vi "Command Drive Distance.vi"(6 "Timeout":dbl=3.0, 8 "Speed":dbl=0.4, 9 "Heading":dbl, 10 "Distance(Feet)":dbl=14.0, 11 "Startup":bool) -> (0 "Angular":dbl, 1 "Reinit":bool, 2 "Linear":dbl, 3 "Completed":bool=TRUE)   [LabVIEW 2019]
uses:
  Command_Execution_State.ctl
  Globals/Sensor_Values.vi
panel:
  in  "Turn Gain":dbl=0.09
  in  "Distance Gain":dbl=0.01
  # "Alpha .06"
  # "Beta .1"
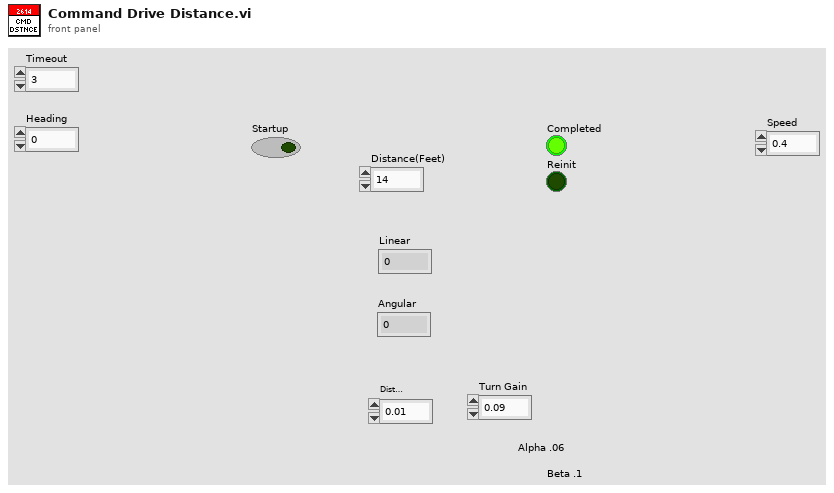
[diagram p1: front panel]
types:
  T1 = typedef "Command_Execution_State.ctl" = enum16{"Initialize", "Execute", "Finish"}
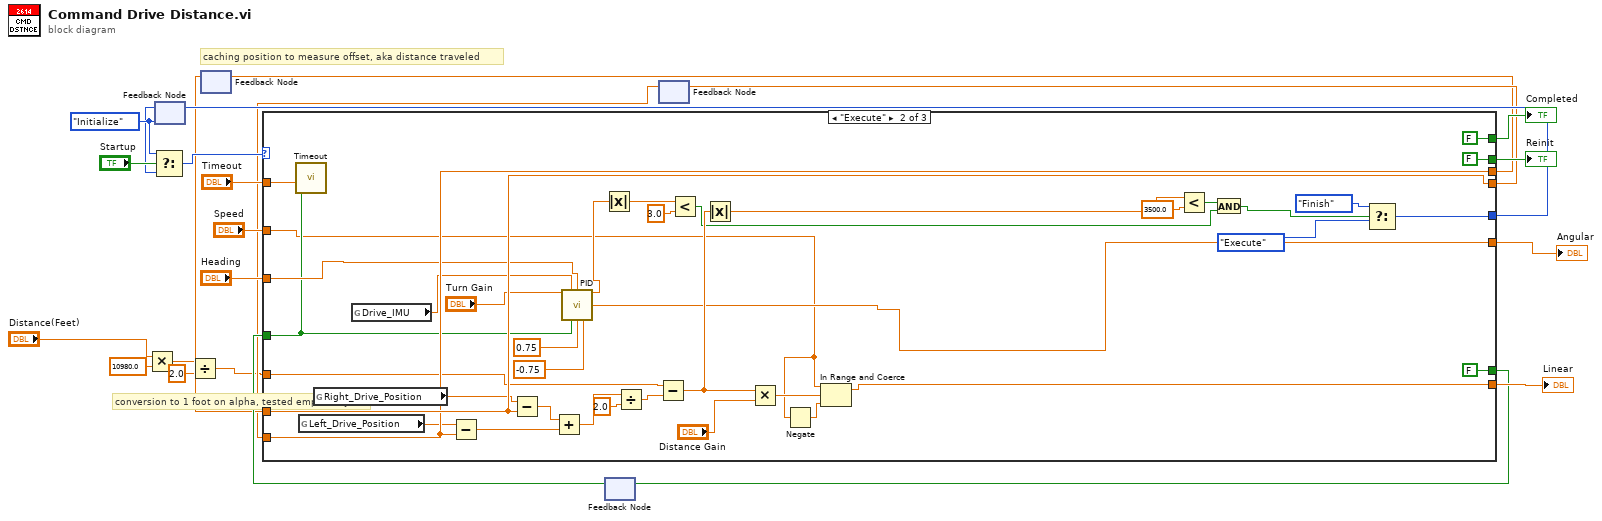
[diagram p0: block diagram]
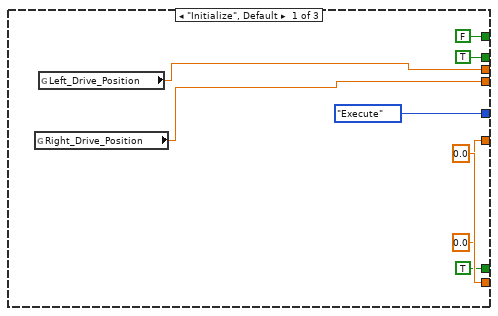
[diagram p2: hidden frame]
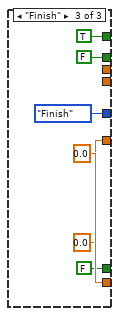
[diagram p3: hidden frame]
diagram:
  w21 = Command_Execution_State."Initialize"
  # "conversion to 1 foot on alpha, tested empirically"
  # "caching position to measure offset, aka distance traveled"
  n1 = Multiply(x="Distance(Feet)", y=10980.0) -> (x*y=w3:dbl)
  n2 = feedback #1(w21) -> (w17:T1)
  n3 = Select(t=w21, s="Startup", f=w17) -> (s? t:f=w22:T1)
  n4 = Divide(x=w3, y=2.0) -> (x/y=w2:dbl)
  n5 = feedback #2() -> (w7:dbl)  [unwired: 1 in]
  n6 = feedback #3() -> (w12:bool)  [unwired: 1 in]
  n7 = feedback #4() -> (w6:dbl)  [unwired: 1 in]
  n8 = case shown="\"Execute\"" w22 {
    tunnel: [FALSE FALSE TRUE] -> w20
    tunnel: [TRUE FALSE FALSE] -> w19
    tunnel: [Command_Execution_State."Execute" w66 Command_Execution_State."Finish"] -> w18
    tunnel: [0.0 ("Left Wheel Velocity") w47 0.0] -> w16
    tunnel: [0.0 ("Right Wheel Velocity") w38 0.0] -> w15
    tunnel: "Heading" -> [_ w40 _]
    tunnel: [TRUE FALSE FALSE] -> w13
    tunnel: w12 -> [_ w39 _]
    tunnel: "Timeout" -> [_ w43 _]
    tunnel: "Speed" -> [_ w34 _]
    tunnel: [w24 w49 _] -> w9
    tunnel: [w25 w48 _] -> w8
    tunnel: w7 -> [_ w49 _]
    tunnel: w6 -> [_ w48 _]
    tunnel: w2 -> [_ w33 _]
    frame "Initialize", Default {
      n9 = global read "Sensor_Values.vi" "Right_Drive_Position"() -> (w24:dbl)
      n10 = global read "Sensor_Values.vi" "Left_Drive_Position"() -> (w25:dbl)
    }
    frame "Execute" {
      n11 = call "Timeout.vi"("Timeout"=w43, "Initialize"=w39) -> ()  [unwired: 1 out]
      n12 = global read "Sensor_Values.vi" "Left_Drive_Position"() -> (w36:dbl)
      n13 = global read "Sensor_Values.vi" "Right_Drive_Position"() -> (w37:dbl)
      n14 = global read "Sensor_Values.vi" "Drive_IMU"() -> (w41:dbl)
      n15 = Subtract(x=w36, y=w48) -> (x-y=w50:dbl)
      n16 = Subtract(x=w37, y=w49) -> (x-y=w52:dbl)
      n17 = Add(x=w52, y=w50) -> (x+y=w53:dbl)
      n18 = call "PID.vi"("Kp"="Turn Gain", "Process Variable"=w41, "Goal"=w40, "Reinit"=w39, "Max Ouput"=0.75, "Min Output"=-0.75) -> ("Current Error"=w42:dbl, "Command"=w38:dbl)  [unwired: 7 in, 1 out]
      n19 = Absolute Value(x=w42) -> (abs(x)=w58:dbl)
      n20 = Divide(x=w53, y=2.0) -> (x/y=w54:dbl)
      n21 = Subtract(x=w33, y=w54) -> (x-y=w64:dbl)
      n22 = Less?(x=w58, y=3.0) -> (x < y?=w57:bool)
      n23 = Absolute Value(x=w64) -> (abs(x)=w65:dbl)
      n24 = Multiply(x=w64, y="Distance Gain") -> (x*y=w62:dbl)
      n25 = Negate(x=w34) -> (-x=w35:dbl)
      n26 = In Range and Coerce(upper limit=w34, x=w62, lower limit=w35) -> (coerced(x)=w47:dbl)  [unwired: 1 out]
      n27 = Less?(x=w65, y=3500.0) -> (x < y?=w60:bool)
      n28 = And(x=w60, y=w57) -> (x .and. y?=w32:bool)
      n29 = Select(t=Command_Execution_State."Finish", s=w32, f=Command_Execution_State."Execute") -> (s? t:f=w66:T1)
    }
    frame "Finish" {
    }
  }
  "Completed" <- w20
  "Reinit" <- w19
  "Linear" <- w16
  "Angular" <- w15
  n30 = feedback-in #1(w18) -> ()
  n31 = feedback-in #2(w8) -> ()
  n32 = feedback-in #3(w13) -> ()
  n33 = feedback-in #4(w9) -> ()
